vi "iWorx New Distance.vi"() -> ()   [LabVIEW 2012]
uses:
  <vilib>/DAQmx/create/channels.llb/DAQmx Create Channel (AO-Voltage-Basic).vi
  <vilib>/DAQmx/create/channels.llb/DAQmx Create Channel (AI-Voltage-Basic).vi
  <vilib>/DAQmx/configure/timing.llb/DAQmx Timing (Sample Clock).vi
  <vilib>/DAQmx/write.llb/DAQmx Write (Analog Wfm 1Chan NSamp).vi
  <vilib>/DAQmx/read.llb/DAQmx Read (Analog Wfm 1Chan NSamp).vi
  <vilib>/measure/mascope.llb/Pulse Measurements 1 chan.vi
  <vilib>/measure/NI_MABase.lvlib
  <vilib>/measure/NI_MAPro.lvlib
panel:
  out "error out":errorcluster
  out "Waveform Chart":dbl(graph)
  in  "Stop Button":bool
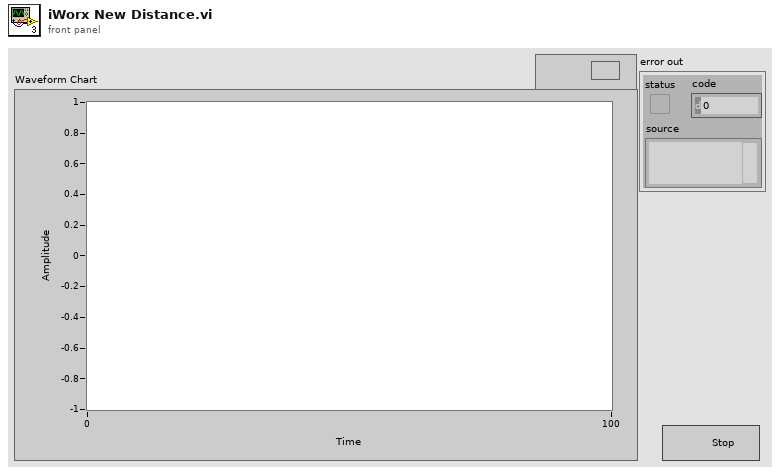
[diagram p1: front panel]
types:
  T1 = enum16{"Sine Wave", "Triangle Wave", "Square Wave", "Sawtooth Wave"}
  T2 = cluster{"high ref level":dbl, "mid ref level":dbl, "low ref level":dbl, "ref units":u16}
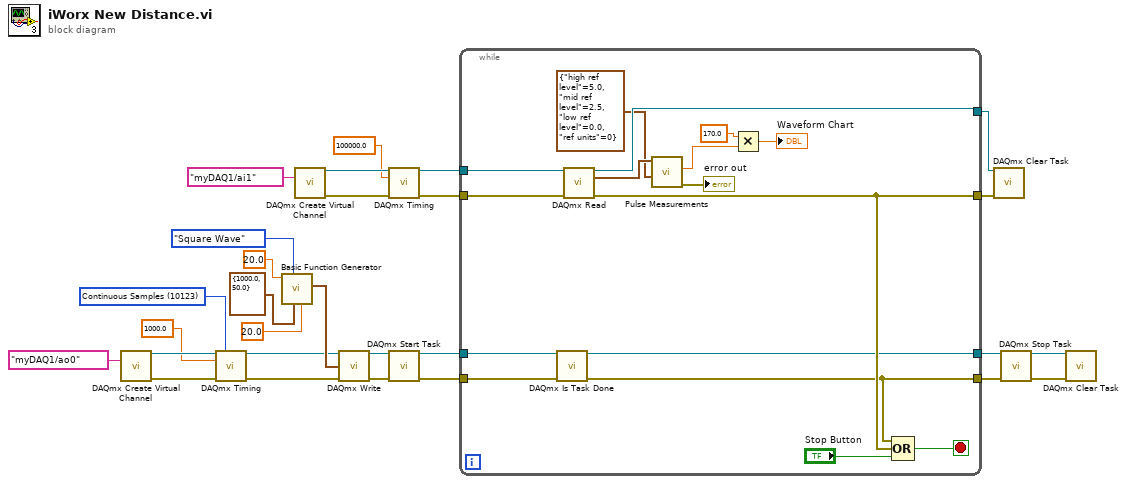
[diagram p0: block diagram]
diagram:
  w14 = 10123 items=["Finite Samples"=10178, "Continuous Samples"=10123, "Hardware Timed Single Point"=12522] ("sample mode")
  n1 = call-poly <vilib>:"DAQmx Create Virtual Channel.vi"("physical channels"=tag "myDAQ1/ao0") -> ("task out"=w28:refnum<k21>, "error out"=w23:errorcluster)  [unwired: 13 in]
  n2 = call-poly <vilib>:"DAQmx Timing.vi"("task/channels in"=w28, "sample mode"=w14, "rate"=1000.0, "error in"=w23) -> ("task out"=w6:refnum<k21>, "error out"=w5:errorcluster)  [unwired: 10 in]
  n3 = call <vilib>:"Basic Function Generator.vi"("square wave duty cycle (%)"=20.0, "sampling info"=cluster{"Fs":dbl, "#s":dbl} {"Fs"=1000.0, "#s"=50.0}, "signal type"=T1."Square Wave", "frequency"=20.0) -> ("signal out"=w10:waveform(dbl))  [unwired: 5 in, 2 out]
  n4 = call-poly <vilib>:"DAQmx Create Virtual Channel.vi"("physical channels"=tag "myDAQ1/ai1") -> ("task out"=w21:refnum<k21>, "error out"=w20:errorcluster)  [unwired: 13 in]
  n5 = call-poly <vilib>:"DAQmx Write.vi"("task/channels in"=w6, "data"=w10, "error in"=w5) -> ("task out"=w8:refnum<k21>, "error out"=w7:errorcluster)  [unwired: 10 in, 1 out]
  n6 = call-poly <vilib>:"DAQmx Timing.vi"("task/channels in"=w21, "rate"=100000.0, "error in"=w20) -> ("task out"=w18:refnum<k21>, "error out"=w17:errorcluster)  [unwired: 11 in]
  n7 = call <vilib>:"DAQmx Start Task.vi"("task/channels in"=w8, "error in"=w7) -> ("task out"=w27:refnum<k21>, "error out"=w24:errorcluster)  [unwired: 12 in]
  n8 = while {
    tunnel: w27 -> [w32]
    tunnel: [w31] -> w4
    tunnel: w24 -> [w29]
    tunnel: [w30] -> w3
    tunnel: w18 -> [w42]
    tunnel: w17 -> [w41]
    tunnel: [w39] -> w16
    tunnel: [w38] -> w15
    stop <- w43 stop-if-true
    n9 = call <vilib>:"DAQmx Is Task Done.vi"("task/channels in"=w32, "error in"=w29) -> ("task out"=w31:refnum<k21>, "error out"=w30:errorcluster)  [unwired: 11 in, 1 out]
    n10 = call-poly <vilib>:"DAQmx Read.vi"("task/channels in"=w42, "error in"=w41) -> ("task out"=w38:refnum<k21>, "data"=w40:waveform(dbl), "error out"=w39:errorcluster)  [unwired: 11 in]
    n11 = call-poly <vilib>:"Pulse Measurements.vi"("reference levels"=T2 {"high ref level"=5.0, "mid ref level"=2.5, "low ref level"=0.0, "ref units"=0}, "signal in"=w40) -> ("error out"=→"error out":errorcluster, "pulse duration"=w37:dbl)  [unwired: 5 in, 3 out]
    n12 = Multiply(x=170.0, y=w37) -> (x*y=→"Waveform Chart":dbl)
    n13 = Compound Arithmetic op=OR(w30, w39, "Stop Button") -> (w43:bool)
  }
  n14 = call <vilib>:"DAQmx Clear Task.vi"("task in"=w15, "error in"=w16) -> ()  [unwired: 13 in, 1 out]
  n15 = call <vilib>:"DAQmx Stop Task.vi"("task/channels in"=w4, "error in"=w3) -> ("task out"=w2:refnum<k21>, "error out"=w1:errorcluster)  [unwired: 12 in]
  n16 = call <vilib>:"DAQmx Clear Task.vi"("task in"=w2, "error in"=w1) -> ()  [unwired: 13 in, 1 out]
